vi "VIE.Module.Queued Message Handler.logEvent.QueuedMessageHandler.vi"(8 "error in (no error)":errorcluster, 9 "Event to Log":string, 10 "QueuedMessageHandler.dqGOOPClass (in)":T1) -> (0 "error out":errorcluster, 2 "QueuedMessageHandler.dqGOOPClass (out)":T1)   [LabVIEW 2010, in "VIE.Module.Queued Message Handler.QueuedMessageHandler.dqGOOPClass.lvlib"]
uses:
  VIE.Module.Queued Message Handler.QueuedMessageHandler.dqGOOPClass.lvlib
  VIE.Module.Queued Message Handler.dqClass_ObjectReference.ctl
  Default.File.ploy.Add Line to Text Log File.File Refnum.vi
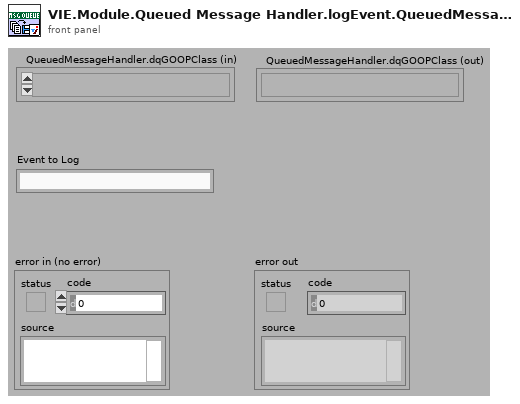
[diagram p1: front panel]
types:
  T1 = typedef "VIE.Module.Queued Message Handler.QueuedMessageHandler.dqGOOPClass.lvlib/VIE.Module.Queued Message Handler.dqClass_ObjectReference.ctl" = refnum<k1>
  T2 = typedef "VIE.Module.Queued Message Handler.QueuedMessageHandler.dqGOOPClass.lvlib/VIE.Module.Queued Message Handler.dqClass_ObjectData.ctl" = cluster{"Message Queue":refnum<queue>, "Log File Refnum":refnum<file>}
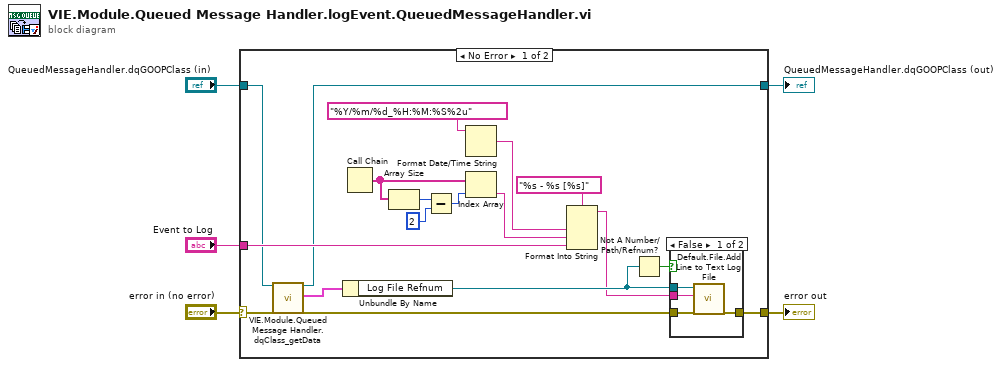
[diagram p0: block diagram]
diagram:
  n1 = case shown="No Error" "error in (no error)" {
    selector: "error in (no error)" -> [w10 w30]
    tunnel: [w23 w30] -> w4
    tunnel: [w7 w29] -> w3
    tunnel: "QueuedMessageHandler.dqGOOPClass (in)" -> [w8 w29]
    tunnel: "Event to Log" -> [w12 _]
    frame No Error {
      n2 = call "VIE.Module.Queued Message Handler.dqClass_getData.vi"("reference"=w8, "error in (no error)"=w10) -> ("duplicate reference"=w7:T1, "data"=w6:T2, "error out"=w9:errorcluster)  [unwired: 14 in, 1 out]
      n3 = Unbundle By Name(w6) -> ("Log File Refnum"=w22:refnum<file>)
      n4 = Call Chain() -> (call chain=w16:string[])
      n5 = Array Size(array=w16) -> (size(s)=w15:i32)
      n6 = Subtract(x=w15, y=2) -> (x-y=w14:i32)
      n7 = Format Date/Time String(time format string (%c)="%Y/%m/%d_%H:%M:%S%2u") -> (date/time string=w20:string)  [unwired: 2 in]
      n8 = Index Array(array=w16, index=w14) -> (element=w11:string)
      n9 = Format Into String(format string="%s - %s [%s]", w20, w11, w12) -> (resulting string=w17:string)  [unwired: 2 in, 1 out]
      n10 = Not A Number/Path/Refnum?(number/path/refnum=w22) -> (NaN/Path/Refnum?=w21:bool)
      n11 = case shown="False" w21 {
        tunnel: w9 -> [w27 w28]
        tunnel: [w26 w28] -> w23
        tunnel: w22 -> [w25 _]
        tunnel: w17 -> [w24 _]
        frame False {
          n12 = call-poly "Default.File.Add Line to Text Log File.vi"("error in (no error)"=w27, "Line to Add"=w24, "File Refnum (in)"=w25) -> ("error out"=w26:errorcluster)  [unwired: 7 in, 1 out]
        }
        frame True {
        }
      }
    }
    frame Error {
    }
  }
  "error out" <- w4
  "QueuedMessageHandler.dqGOOPClass (out)" <- w3
